vi "(SubVI)Serial_COM port Check.vi"(7 "Auto Detect?":bool, 8 "error in (no error)":errorcluster caption="에러 입력(에러 없음)", 9 "ID to Exclude":u8 format="%.0x", 10 "ID to Find":u8 format="%.0x", 11 "VISA resource name":refnum<visa-resource-name>) -> (0 "error out":errorcluster caption="에러 출력", 1 "IC Type":T2, 2 "BD Version":T1 {"BD FW Version" format="%08x"}, 3 "VISA resource name out":refnum<visa-resource-name>, 4 "I2C Slave ID":cluster{string, u8}[](array[cluster]), 5 "BD Info Str":string, 6 "Default I2C Slave ID":u8)   [LabVIEW 2020]
uses:
  Libraries/Haptic IC Class/Haptic IC/Controls/(Ctrl)IC Type.ctl
  Controls/(Ctrl)Serial_FGV Function.ctl
  3574bd08-2314-4aeb-a6ee-42674643e89d.vi
  <vilib>/Comparison/Equal/Equal Functor/Equal Functor.lvclass
  <vilib>/Instr/_visa.llb/VISA Find Search Mode.ctl
  5283ad07-9809-4087-83e9-a87157ce31b4.vi
  Libraries/Haptic IC Class/Haptic IC/Haptic IC.lvclass
panel:
  # "(SubVI)Serial_COM port Check.vi By hspark\n\nDescription : VISA Serial 연결 후 Board Information 명령어로 Board HW Version, FW Version, Chip ID 리스트 등을 얻는 VI\n\nInput : \n1. VISA resource name : 사용자가 선택한 COM port\n2. Auto Detect? : True 입력 시 VISA resource name 입력을 무시하고 PC에 연결되어 있는 모든 COM port에 대해 Checking 진행\n                        순차적으로 진행 중 Board를 찾으면 중지함\n3. ID to Find : 9786 등과 같이 Chip ID 확인이 불가능한 IC의 경우, 찾으려는 ID를 입력받아서 ID List에 있는 경우 해당 ID가 선택되게 함\n\nOutput : \n1. VISA resource name out : 연결된 COM port 출력\n2. BD FW Version : U32로 된 Board의 FW Version\n3. BD HW Version : 프로토콜에 명시된 Board의 HW Version (모델 추가 시 열거형 타입 정의 업데이트)\n4. I2C Slave ID : Board로부터 수신받은 I2C Slave ID 목록. 링 컨트롤 업데이트를 위한 클러스터 배열 출력.\n5. Default I2C Slave ID : Chip ID가 있는 첫번째 Slave ID. 모든 Slave가 Chip ID가 없는 경우 첫번째 Slave ID\n\nLabVIEW Version : 2020 SP1 이상\n\nNote :\n\nUpdate : 2021.12.20"
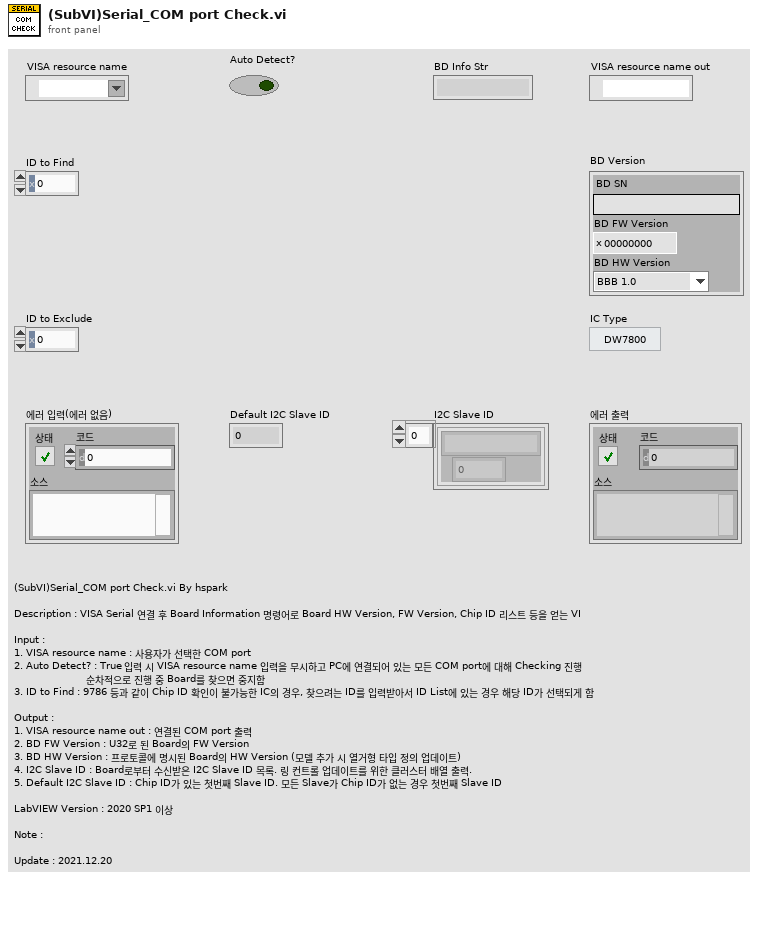
[diagram p1: front panel]
types:
  T1 = cluster{"BD SN":string, "BD FW Version":u32, "BD HW Version":enum8{"BBB 1.0", "BBB 1.1", "WBB 1.0", "reserved", "RedNoah3"}}
  T2 = typedef "Haptic IC.lvclass/(Ctrl)IC Type.ctl" = enum8{"DW7800", "DW7802", "DW7912", "DW7914"}
  T3 = typedef "(Ctrl)Serial_FGV Function.ctl" = enum16{"Initialize", "Read", "Read All", "Write", "Flush Buffer", "Get Ref.", "Close"}
  T4 = typedef "VISA Find Search Mode.ctl" = u32
  T5 = enum8{"BBB 1.0", "BBB 1.1", "WBB 1.0", "reserved", "RedNoah3"}
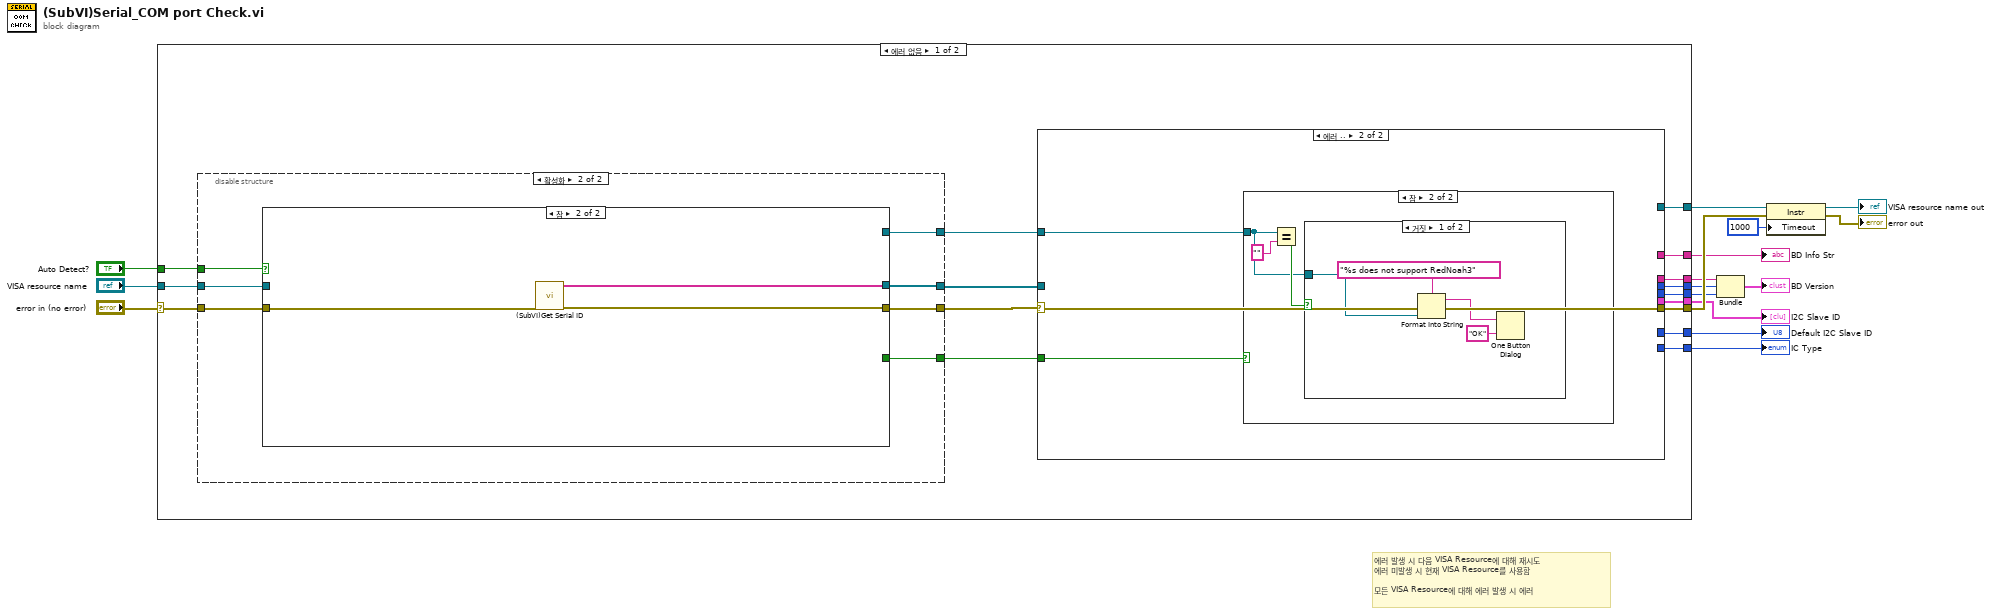
[diagram p0: block diagram]
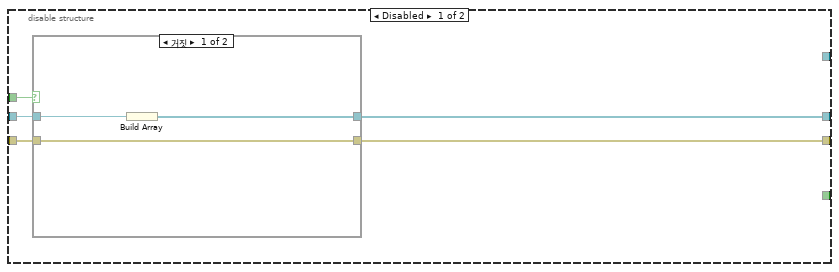
[diagram p2: hidden frame]
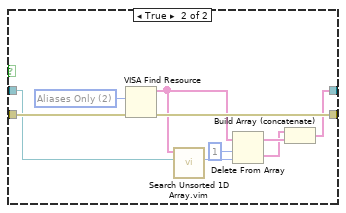
[diagram p3: hidden frame]
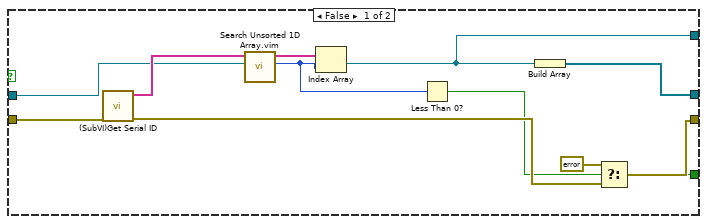
[diagram p4: hidden frame]
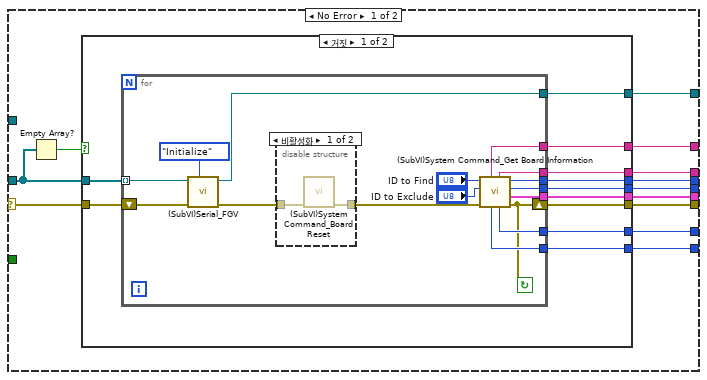
[diagram p5: hidden frame]
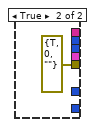
[diagram p7: hidden frame]
diagram:
  # "에러 발생 시 다음 VISA Resource에 대해 재시도\n에러 미발생 시 현재 VISA Resource를 사용함 \n\n모든 VISA Resource에 대해 에러 발생 시 에러"
  n1 = case shown="에러 없음" "error in (no error)" {
    selector: "error in (no error)" -> [w32 w124]
    tunnel: [w31 w124] -> w15
    tunnel: [w30 _] -> w3
    tunnel: [w29 _] -> w4
    tunnel: "Auto Detect?" -> [w28 _]
    tunnel: "VISA resource name" -> [w27 w123]
    tunnel: [w26 _] -> w12
    tunnel: [w25 _] -> w11
    tunnel: [w24 w123] -> w8
    tunnel: [w23 _] -> w10
    tunnel: [w22 _] -> w5
    tunnel: [w21 _] -> w1
    frame No Error {
      n2 = disable-structure shown="활성화" {
        disable-tunnel: w32 -> [w37 w57]
        disable-tunnel: w28 -> [w36 w55]
        disable-tunnel: w27 -> [w35 w54]
        disable-tunnel: [w34 w56] -> w20
        disable-tunnel: [w33 w53] -> w19
        disable-tunnel: [_ w52] -> w18
        disable-tunnel: [_ w51] -> w17
        frame Disabled {
          n3 = case shown="거짓" w36 {
            tunnel: w35 -> [w40 w47]
            tunnel: [w39 w41] -> w33
            tunnel: w37 -> [w38 w49]
            tunnel: [w38 w48] -> w34
            frame False {
              n4 = Build Array(w40) -> (w39:refnum<visa-resource-name>[])
            }
            frame True {
              w50 = T4 2 items=["Canonical Names Only"=0, "Aliases Only"=2, "Include Matching Aliases"=3, "Include All Aliases"=4] ("Search Mode")
              n5 = VISA Find Resource(8:w49, 10:w50) -> (0:w48:errorcluster, 3:w46:string[])  [unwired: 1 in, 1 out]
              n6 = call "Search Unsorted 1D Array.vim"("element"=w47, "unsorted 1D array"=w46) -> ("index of element"=w45:i32)  [unwired: 9 in]
              n7 = Delete From Array(array=w46, length=1 ("길이"), index=w45) -> (deleted portion=w42:string[], array with subset deleted=w43:string[])
              n8 = Build Array (concatenate)(w42, w43) -> (w41:string[])
            }
          }
        }
        frame Enabled {
          n9 = case shown="참" w55 {
            tunnel: w57 -> [w66 w69]
            tunnel: [w60 w68] -> w56
            tunnel: w54 -> [w58 _]
            tunnel: [w64 w67] -> w53
            tunnel: [w59 _] -> w52
            tunnel: [w58 _] -> w51
            frame False {
              n10 = call "(SubVI)Get Serial ID.vi"("error in (no error)"=w66) -> ("error out"=w62:errorcluster, "port"=w65:string[])  [unwired: 9 in]
              n11 = call "Search Unsorted 1D Array.vim"("element"=w58, "unsorted 1D array"=w65) -> ("index of element"=w63:i32)  [unwired: 9 in]
              n12 = Index Array(array=w65, index=w63) -> ()  [unwired: 1 out]
              n13 = Less Than 0?(x=w63) -> (x < 0?=w59:bool)
              n14 = Build Array(w58) -> (w64:refnum<visa-resource-name>[])
              n15 = Select(t=errorcluster {"status"=TRUE, "code"=0, "source"=""}, s=w59, f=w62) -> (s? t:f=w60:errorcluster)
            }
            frame True {
              n16 = call "(SubVI)Get Serial ID.vi"("error in (no error)"=w69) -> ("error out"=w68:errorcluster, "port"=w67:string[])  [unwired: 9 in]
            }
          }
        }
      }
      n17 = case shown="에러 .." w20 {
        selector: w20 -> [w81 w115]
        tunnel: [w80 w115] -> w31
        tunnel: [w79 _] -> w30
        tunnel: [w78 _] -> w29
        tunnel: [w77 _] -> w26
        tunnel: [w76 _] -> w25
        tunnel: [w75 _] -> w24
        tunnel: [w74 _] -> w23
        tunnel: [w73 _] -> w22
        tunnel: [w72 _] -> w21
        tunnel: w19 -> [w71 _]
        tunnel: w18 -> [_ w113]
        tunnel: w17 -> [_ w114]
        frame No Error {
          n18 = Empty Array?(array=w71) -> (empty?=w70:bool)
          n19 = case shown="거짓" w70 {
            tunnel: w81 -> [w92 _]
            tunnel: [w91 errorcluster {"status"=TRUE, "code"=0, "source"=""} ("error IO")] -> w80
            tunnel: [w90 _] -> w79
            tunnel: [w89 _] -> w78
            tunnel: [w88 _] -> w77
            tunnel: [w87 _] -> w76
            tunnel: [w86 _] -> w75
            tunnel: [w85 _] -> w74
            tunnel: [w84 _] -> w73
            tunnel: [w83 _] -> w72
            tunnel: w71 -> [w82 _]
            frame False {
              n20 = for {
                tunnel: [w107] -> w90
                tunnel: [w106] -> w89
                tunnel: [w105] -> w88
                tunnel: [w104] -> w87
                tunnel: [w103] -> w86
                tunnel: [w102] -> w85
                tunnel: [w101] -> w84
                tunnel: [w100] -> w83
                tunnel: w82 -> [w98] mode=indexing
                shift-right: [w93] -> w91
                shift-left: w92 -> [w108]
                stop <- w93 continue-if-true
                n21 = call "(SubVI)Serial_FGV.vi"("Function"=(Ctrl)Serial_FGV_Function."Initialize", "error in (no error)"=w108, "VISA resource name"=w98) -> ("error out"=w94:errorcluster, "VISA resource name out"=w103:refnum<visa-resource-name>)  [unwired: 6 in, 1 out]
                n22 = disable-structure shown="비활성화" {
                  disable-tunnel: w94 -> [w110 w111]
                  disable-tunnel: [w109 w111] -> w95
                  frame Disabled {
                    n23 = call "(SubVI)System Command_Board Reset.vi"("error in (no error)"=w110) -> ("error out"=w109:errorcluster)  [unwired: 9 in, 1 out]
                  }
                  frame Enabled {
                  }
                }
                n24 = call "(SubVI)System Command_Get Board Information.vi"("error in (no error)"=w95, "ID to Exclude"="ID to Exclude", "ID to Find"="ID to Find") -> ("error out"=w93:errorcluster, "I2C Slave ID"=w105:cluster{string, u8}[], "BD HW Version"=w107:T5, "BD FW Version"=w106:u32, "Default I2C Slave ID"=w104:u8, "BD SN"=w100:string, "IC Type"=w101:T2, "BD Info Str"=w102:string)  [unwired: 1 in]
              }
            }
            frame True {
            }
          }
        }
        frame Error {
          n25 = case shown="참" w113 {
            tunnel: w114 -> [_ w116]
            frame False {
            }
            frame True {
              n26 = Equal?(x=w116, y="") -> (x = y?=w117:bool)
              n27 = case shown="거짓" w117 {
                tunnel: w116 -> [w122 _]
                frame False {
                  n28 = Format Into String(format string="%s does not support RedNoah3" ("포맷 문자열"), w122) -> (resulting string=w120:string)  [unwired: 2 in, 1 out]
                  n29 = One Button Dialog(message=w120, button name ("OK")="OK" ("버튼 이름(\"확인\")")) -> ()  [unwired: 1 out]
                }
                frame True {
                }
              }
            }
          }
        }
      }
    }
    frame Error {
    }
  }
  "I2C Slave ID" <- w12
  "Default I2C Slave ID" <- w11
  "BD Info Str" <- w10
  "IC Type" <- w5
  n30 = Bundle("BD SN"=w1, "BD FW Version"=w4, "BD HW Version"=w3) -> (→"BD Version":T1)  [unwired: 1 in]
  n31 = property class="Instr"(reference=w8, error in=w15, "Timeout"=u32 1000 ("General Settings:Timeout Value")) -> (reference out=→"VISA resource name out":refnum<visa-resource-name>, error out=→"error out":errorcluster)
